vi "trace_extra2.vi"(2 "Extra trace 1":sgl[](array[numeric]), 3 "Extra trace 0":sgl[](array[numeric])) -> ()   [LabVIEW 2011]
panel:
  # "Supply data to be added to the trace in the \"Trace data 0\", \"Trace data 1\".   Each is reshaped to be a 3-vector"
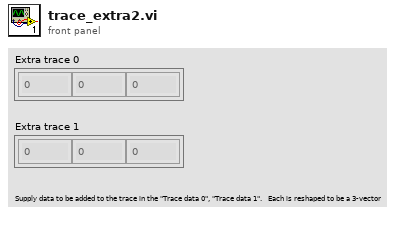
[diagram p1: front panel]
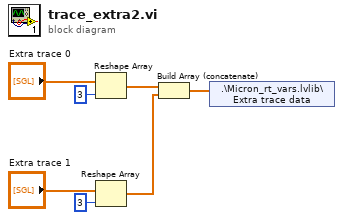
[diagram p0: block diagram]
diagram:
  n1 = Reshape Array("Extra trace 0", 3 ("dimension size")) -> (w2:sgl[])
  n2 = Reshape Array("Extra trace 1", 3 ("dimension size")) -> (w3:sgl[])
  n3 = Build Array (concatenate)(w2, w3) -> (w1:sgl[])
  n4 = shared-variable ".\\Micron_rt_vars.lvlib\\Extra trace data"(w1) -> ()  [unwired: 2 out]
